vi "Should Have Error.vi"() -> (2 "Pass?":bool)   [LabVIEW 2014]
uses:
  Launch.lvclass
  <vilib>/ActorFramework/Message Queue/Message Queue.lvclass/Message Queue.ctl
  <vilib>/ActorFramework/Actor/Actor.lvclass
  <vilib>/ActorFramework/Message Queue/Message Queue.lvclass
panel:
  out "error out":errorcluster
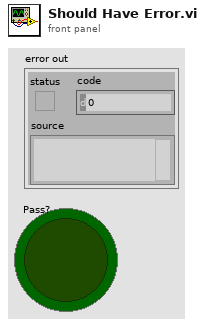
[diagram p1: front panel]
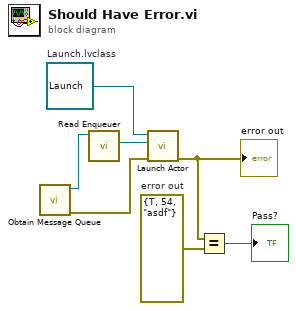
[diagram p0: block diagram]
diagram:
  w5 = errorcluster {"status"=TRUE, "code"=54, "source"="asdf"}  # error out
  w7 = refnum<class "Launch.lvclass"> refnum  # Launch.lvclass
  n1 = call <vilib>:"Obtain Message Queue.vi"() -> ("error out"=w3:errorcluster, "Message Queue"=w2:refnum<class "Message Queue.lvclass">)  [unwired: 10 in]
  n2 = call <vilib>:"Read Enqueuer.vi"("Message Queue"=w2) -> ("Message Enqueuer"=w1:refnum<class "Message Enqueuer.lvclass">)  [unwired: 10 in]
  n3 = call <vilib>:"Launch Actor.vi"("error in (no error)"=w3, "Actor-to-Caller Enqueuer"=w1, "Actor"=w7) -> ("error out"=w6:errorcluster)  [unwired: 7 in, 1 out]
  "error out" <- w6
  n4 = Equal?(x=w6, y=w5) -> (x = y?=→"Pass?":bool)
